vi "logrecordnumber.vi"(7 "logsetting":enum16{"error", "info", "debug"}(ring), 8 "error in":errorcluster, 9 "logtype":enum16{"error", "info", "debug"}(ring), 10 "LogPath":path, 11 "Msg":dbl) -> (0 "error out":errorcluster)   [LabVIEW 2011]
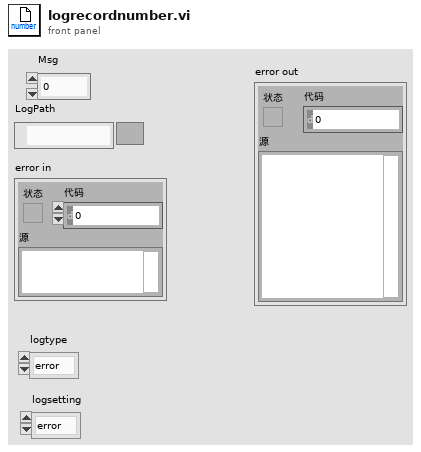
[diagram p1: front panel]
types:
  T1 = enum16{"open", "replace", "create", "open or create", "replace or create", "replace or create with confirmation"}
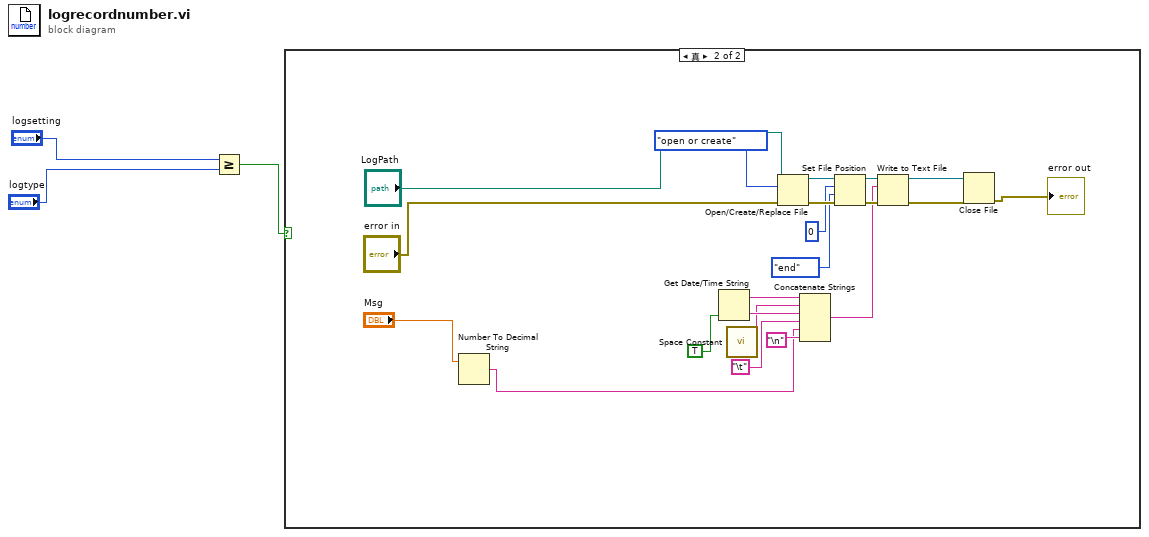
[diagram p0: block diagram]
diagram:
  n1 = Greater Or Equal?(x="logsetting", y="logtype") -> (x >= y?=w1:bool)
  n2 = case shown="真" w1 {
    frame False {
    }
    frame True {
      n3 = Number To Decimal String(number="Msg") -> (decimal integer string=w4:string)  [unwired: 1 in]
      n4 = Get Date/Time String(want seconds? (F)=TRUE ("需要秒？(F)")) -> (date string=w10:string, time string=w12:string)  [unwired: 2 in]
      n5 = call <vilib>:"Space Constant.vi"() -> ("String"=w11:string)
      n6 = Open/Create/Replace File(file path (use dialog)="LogPath", error in="error in", operation (0:open)=T1."open or create" ("操作(0:open)")) -> (refnum out=w6:refnum<file>, error out=w17:errorcluster)  [unwired: 3 in, 1 out]
      n7 = Concatenate Strings(w10, w11, w12, "\t", w4, "\n") -> (w15:string)
      n8 = Set File Position(offset (in bytes) (0)=i64 0 ("偏移量（字节）（0）"), refnum=w6, from (0:start)=enum16{"start", "end", "current"}."end" ("自（0:起始）"), error in=w17) -> (refnum out=w8:refnum<file>, error out=w18:errorcluster)
      n9 = Write to Text File(file (use dialog)=w8, text=w15, error in=w18) -> (refnum out=w20:refnum<file>, error out=w21:errorcluster)  [unwired: 1 in, 1 out]
      n10 = Close File(refnum=w20, error in=w21) -> (error out=→"error out":errorcluster)  [unwired: 1 out]
    }
  }
